vi "Tetra_RX-PROD_Close.vi"() -> (0 "error out":errorcluster={"status"=FALSE, "code"=1073676418, "source"="VISA Close in Tetra_RX-PROD_Close.vi"}, 2 "Status":string="Setting up Power Supplies...ERROR!...\rDone !!!\n...Shut Off RF\rDONE!!!")   [LabVIEW 2018]
uses:
  <vilib>/Utility/error.llb/DialogType.ctl
  Infrastructure/Test Parameter Globals_1.0.0.vi
  Initialize References/Station References Global.vi
  Tetra_Globals.vi
  Instruments/Keysight N6700/Agilent N6700 Series/Agilent N6700 Series.lvlib
  Instruments/PNA/lib functions/Agilent ENA Series.lvlib
panel:
  out "Capture RxData":bool
  out "DeleteDir(t)":bool
  out "ZipCaptures(t)":bool
  out "stripped path":path=path "C:/RageATE Results/REV-B_TETRA_RX-PROD/5_25_2022/REV-B_TETRA_RX-PROD_SN_ RGE2100033_052522-171445_RxCaptureFiles - Copy"
  in  "close serial(t)":bool=TRUE
  in  "Close Oven(t)":bool=TRUE
  out "Use PS1-2":bool=TRUE
  out "PS1-2(A)":dbl
  out "PS1-2(V)":dbl=1000000.0
  out "Use PS1-1":bool=TRUE
  out "Text":refnum<vi>
  in  "Close  PNA (T)":bool=TRUE
  in  "Close Power Supply (T)":bool=TRUE
  in  "error in (no error)":errorcluster
  out "PS1-1(A)":dbl
  out "PS1-1(V)":dbl=3.0
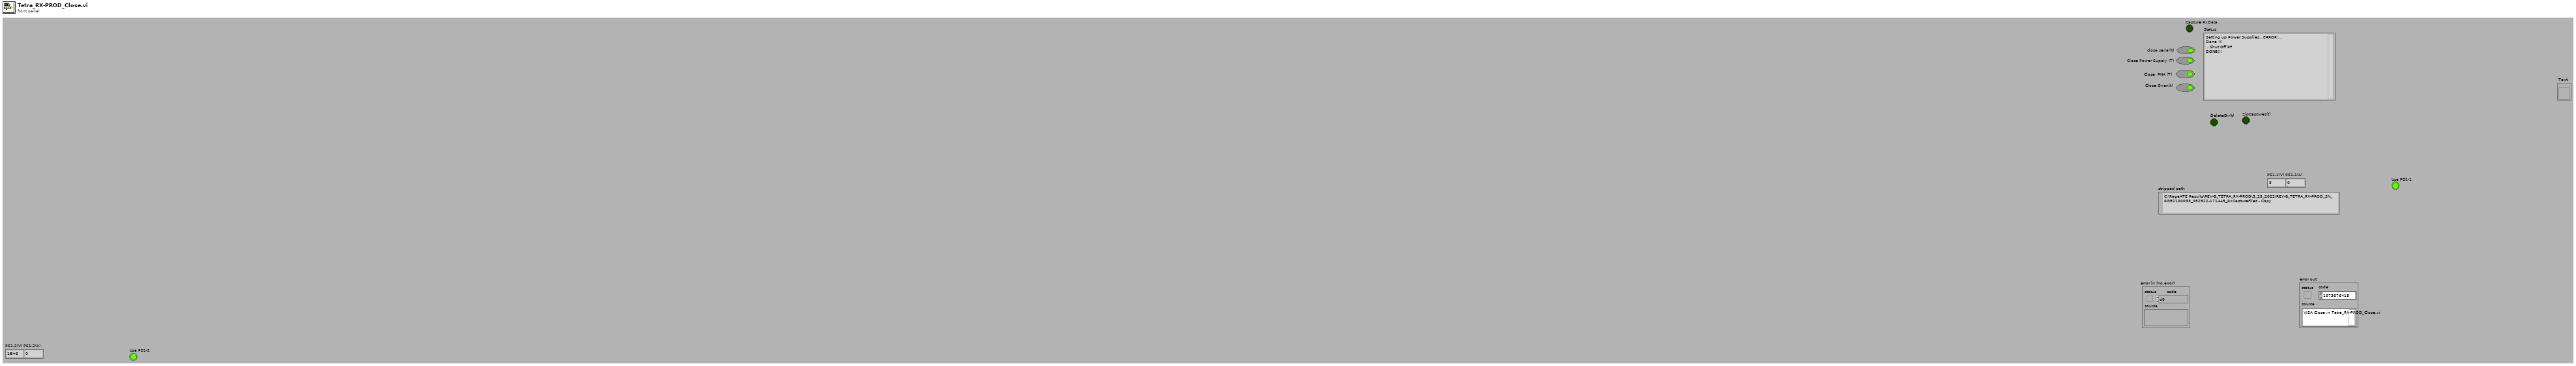
[diagram p1: front panel]
types:
  T1 = typedef "DialogType.ctl" = u16
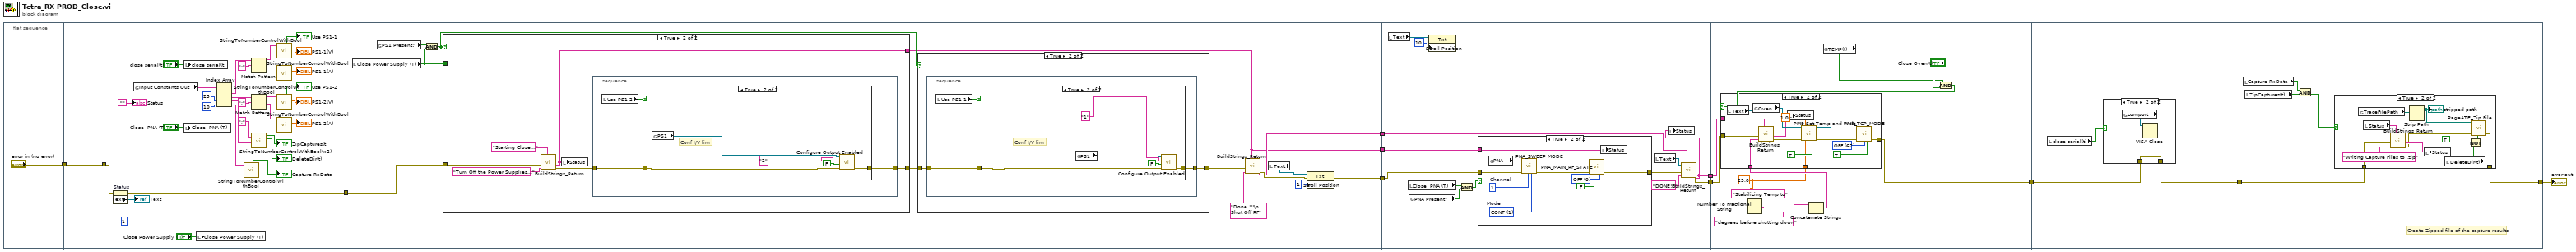
[diagram p0: block diagram]
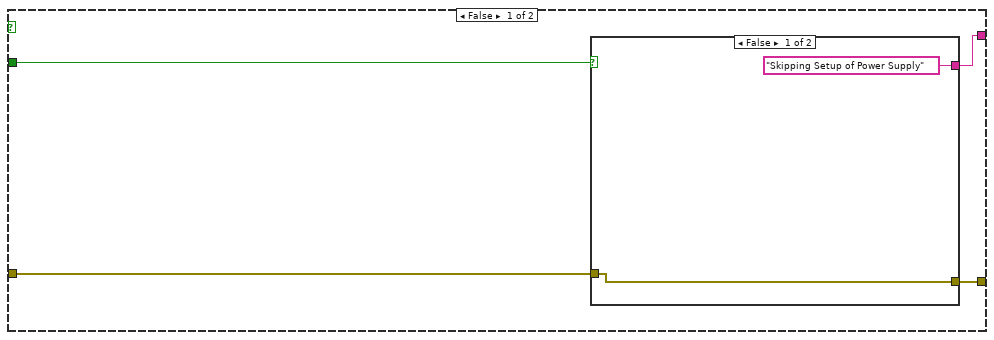
[diagram p4: hidden frame]
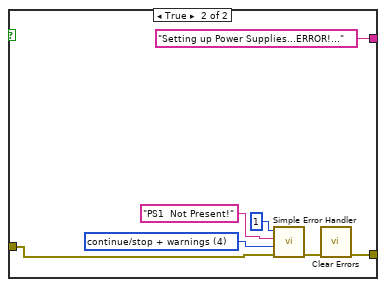
[diagram p5: hidden frame]
diagram:
  n1 = flat-sequence {
    tunnel: ["error in (no error)"] -> w5
    tunnel: w5 -> [w13]
    tunnel: [w13] -> w4
    tunnel: [w33] -> w10
    tunnel: w4 -> [w23]
    tunnel: [w56] -> w6
    tunnel: w10 -> [w52]
    tunnel: [w45] -> w3
    tunnel: [w44] -> w2
    tunnel: [w99] -> w7
    tunnel: [w108] -> w9
    tunnel: w6 -> [w102]
    tunnel: w3 -> [w100]
    tunnel: w2 -> [w98]
    tunnel: w9 -> [w128]
    tunnel: [w123] -> w8
    tunnel: w7 -> [w127]
    tunnel: w8 -> [w150]
    tunnel: [w149] -> w1
    tunnel: [w157] -> w11
    tunnel: w1 -> [w158]
    frame #0 {
    }
    frame #1 {
    }
    frame #2 {
      (unwired) u32 1 ("Text.Scroll Position")
      n2 = property on="Status" class="Str"(error in=w23) -> (error out=w33:errorcluster, "Text"=→"Text":refnum<vi>)  [unwired: 1 in, 1 out]
      n3 = global read "Test Parameter Globals_1.0.0.vi" "Input Constants Out"() -> (w24:string[])
      n4 = local write "close serial(t)"("close serial(t)") -> ()
      n5 = local write "Close  PNA (T)"("Close  PNA (T)") -> ()
      n6 = local write "Close Power Supply (T)"("Close Power Supply (T)") -> ()
      n7 = Index Array(array=w24, index #3=25 ("index"), index #4=10 ("index")) -> (element #1=w32:string, element #2=w25:string, element #3=w20:string, element #4=w15:string)  [unwired: 2 in]
      n8 = call "StringToNumberControlWithBool.vi"("String In"=w15) -> ("NOT = 0"=→"Capture RxData":bool)  [unwired: 7 in, 1 out]
      n9 = Match Pattern(string=w32, regular expression=";") -> (before substring=w38:string, after substring=w37:string)  [unwired: 1 in, 2 out]
      n10 = Match Pattern(string=w25, regular expression=";") -> (before substring=w30:string, after substring=w29:string)  [unwired: 1 in, 2 out]
      n11 = call "StringToNumberControlWithBool(x2).vi"("Seperator"=";", "string"=w20) -> ("NOT_0(2)"=→"DeleteDir(t)":bool, "NOT_0?"=→"ZipCaptures(t)":bool)  [unwired: 3 in, 5 out]
      n12 = call "StringToNumberControlWithBool.vi"("String In"=w38) -> ("Number Out"=→"PS1-1(V)":dbl, "NOT = 0"=→"Use PS1-1":bool)  [unwired: 7 in]
      n13 = call "StringToNumberControlWithBool.vi"("String In"=w37) -> ("Number Out"=→"PS1-1(A)":dbl)  [unwired: 7 in, 1 out]
      n14 = call "StringToNumberControlWithBool.vi"("String In"=w30) -> ("Number Out"=→"PS1-2(V)":dbl, "NOT = 0"=→"Use PS1-2":bool)  [unwired: 7 in]
      n15 = call "StringToNumberControlWithBool.vi"("String In"=w29) -> ("Number Out"=→"PS1-2(A)":dbl)  [unwired: 7 in, 1 out]
      "Status" <- ""
    }
    frame #3 {
      n16 = local read "Close Power Supply (T)"() -> (w46:bool)
      n17 = global read "Station References Global.vi" "PS1 Present?"() -> (w51:bool)
      n18 = And(x=w51, y=w46) -> (x .and. y?=w48:bool)
      n19 = case shown="True" w48 {
        tunnel: [w72 w83] -> w49
        tunnel: w52 -> [w71 w85]
        tunnel: [w70 w82] -> w44
        tunnel: w46 -> [w69 _]
        frame False {
          n20 = case shown="False" w69 {
            tunnel: [w74 w77] -> w72
            tunnel: w71 -> [w74 w76]
            tunnel: ["Skipping Setup of Power Supply" "Setting up Power Supplies...ERROR!..."] -> w70
            frame False {
            }
            frame True {
              w79 = T1 4 items=["no dialog", "OK message", "continue or stop message", "OK message + warnings", "continue/stop + warnings"] ("type of dialog (OK msg:1)")
              n21 = call <vilib>:"Simple Error Handler.vi"("error code (no error:0)"=1, "error source (\" \")"="PS1  Not Present!" ("error source (\" \")"), "type of dialog (OK msg:1)"=w79, "error in (no error)"=w76) -> ("error out"=w78:errorcluster)  [unwired: 1 in, 4 out]
              n22 = call <vilib>:"Clear Errors.vi"("error in (no error)"=w78) -> ("error out"=w77:errorcluster)  [unwired: 5 in, 1 out]
            }
          }
        }
        frame True {
          n23 = call "BuildStrings_Return.vi"("Input String"="Starting Close...", "New String"="Turn Off the Power Supplies...", "error in (no error)"=w85) -> ("error out"=w84:errorcluster, "concatenated string"=w82:string)  [unwired: 6 in, 1 out]
          n24 = local write "Status"(w82) -> ()
          n25 = stacked-sequence {
            tunnel: w84 -> [w90]
            tunnel: [w88] -> w83
            frame #0 {
              n26 = local read "Use PS1-2"() -> (w89:bool)
              n27 = case shown="True" w89 {
                tunnel: [w91 w94] -> w88
                tunnel: w90 -> [w91 w93]
                frame False {
                }
                frame True {
                  # "Conf I/V lim"
                  n28 = global read "Station References Global.vi" "PS1"() -> (w92:refnum<visa-resource-name>)
                  n29 = call "Configure Output Enabled.vi"("error in (no error)"=w93, "Enable Output (False)"=FALSE, "Channel Name (1)"="2", "VISA resource name"=w92) -> ("error out"=w94:errorcluster)  [unwired: 6 in, 1 out]
                }
              }
            }
          }
        }
      }
      n30 = case shown="True" w48 {
        tunnel: [w57 w59] -> w47
        tunnel: w49 -> [w57 w58]
        frame False {
        }
        frame True {
          n31 = stacked-sequence {
            tunnel: w58 -> [w62]
            tunnel: [w60] -> w59
            frame #0 {
              n32 = local read "Use PS1-1"() -> (w61:bool)
              n33 = case shown="True" w61 {
                tunnel: [w63 w66] -> w60
                tunnel: w62 -> [w63 w65]
                frame False {
                }
                frame True {
                  # "Conf I/V lim"
                  n34 = global read "Station References Global.vi" "PS1"() -> (w64:refnum<visa-resource-name>)
                  n35 = call "Configure Output Enabled.vi"("error in (no error)"=w65, "Enable Output (False)"=FALSE, "Channel Name (1)"="1", "VISA resource name"=w64) -> ("error out"=w66:errorcluster)  [unwired: 6 in, 1 out]
                }
              }
            }
          }
        }
      }
      n36 = call "BuildStrings_Return.vi"("Input String"=w44, "New String"="Done !!!\n...Shut Off RF", "error in (no error)"=w47) -> ("error out"=w53:errorcluster, "concatenated string"=w45:string)  [unwired: 6 in, 1 out]
      n37 = local read "Text"() -> (w55:refnum<vi>)
      n38 = property class="Txt"(reference=w55, error in=w53, "Scroll Position"=u32 1) -> (error out=w56:errorcluster)  [unwired: 1 out]
    }
    frame #4 {
      n39 = local read "Text"() -> (w106:refnum<vi>)
      n40 = local read "Close  PNA (T)"() -> (w105:bool)
      n41 = global read "Station References Global.vi" "PNA Present?"() -> (w104:bool)
      n42 = property class="Txt"(reference=w106, "Scroll Position"=u32 10) -> ()  [unwired: 1 in, 2 out]
      n43 = And(x=w105, y=w104) -> (x .and. y?=w103:bool)
      n44 = case shown="True" w103 {
        tunnel: w102 -> [w110 w118]
        tunnel: [w110 w116] -> w101
        tunnel: w98 -> [_ w111]
        frame False {
        }
        frame True {
          w113 = 0 items=["OFF", "ON"] ("STATE(0=OFF)")
          w119 = 1 items=["HOLD", "CONT", "GROUP", "SINGLE"]  # Mode
          w120 = 1  # Channel
          n45 = global read "Station References Global.vi" "PNA"() -> (w117:refnum<visa-resource-name>)
          n46 = call "PNA_SWEEP MODE.vi"("Mode"=w119, "Channel"=w120, "error in (no error)"=w118, "VISA resource name"=w117) -> ("error out"=w115:errorcluster, "VISA resource name out"=w114:refnum<visa-resource-name>)  [unwired: 6 in]
          n47 = call "PNA_MAIN_RF_STATE.vi"("Session In"=w114, "error in"=w115, "RO(T)"=FALSE, "STATE(0=OFF)"=w113) -> ("error out"=w116:errorcluster)  [unwired: 9 in, 2 out]
          n48 = local write "Status"(w111) -> ()
        }
      }
      n49 = local read "Text"() -> (w97:refnum<vi>)
      n50 = call "BuildStrings_Return.vi"("Input String"=w100, "New String"="DONE!!!", "error in (no error)"=w101, "reference"=w97) -> ("error out"=w108:errorcluster, "concatenated string"=w99:string)  [unwired: 5 in, 1 out]
      n51 = local write "Status"(w99) -> ()
    }
    frame #5 {
      w121 = 25.0 ("Set Point")
      n52 = Number To Fractional String(number=w121) -> (F-format string=w122:string)  [unwired: 3 in]
      n53 = Concatenate Strings("Stabilizing Temp to" ("New String"), w122, "degrees before shutting down" ("string")) -> (w126:string)
      n54 = global read "Tetra_Globals.vi" "TEMP(t)"() -> (w125:bool)
      n55 = And(x=w125, y="Close Oven(t)") -> (x .and. y?=w124:bool)
      n56 = case shown="True" w124 {
        tunnel: w128 -> [w132 w144]
        tunnel: w127 -> [_ w146]
        tunnel: w126 -> [_ w145]
        tunnel: [w132 w137] -> w123
        tunnel: w121 -> [_ w134]
        frame False {
        }
        frame True {
          w139 = u16 62 items=["READ ONLY"=0, "AUTO"=10, "OFF"=62, "MAN"=54] ("MODE")
          n57 = local read "Text"() -> (w135:refnum<vi>)
          n58 = global read "Station References Global.vi" "Oven"() -> (w147:refnum<visa-resource-name>)
          n59 = call "BuildStrings_Return.vi"("Input String"=w146, "New String"=w145, "error in (no error)"=w144, "reference"=w135) -> ("error out"=w143:errorcluster, "concatenated string"=w141:string)  [unwired: 5 in, 1 out]
          n60 = local write "Status"(w141) -> ()
          n61 = call "PM9 Set Temp and Wait.vi"("VISA"=w147, "Error In"=w143, "Accuracy +/-"=1.0, "Set Point"=w134, "close session(t)"=TRUE) -> ("visa"=w136:refnum<visa-resource-name>, "error out"=w140:errorcluster)  [unwired: 11 in, 2 out]
          n62 = call "PM9_TCP_MODE.vi"("VISA"=w136, "error in (no error)"=w140, "MODE"=w139, "Close tcp(t)"=TRUE) -> ("error out"=w137:errorcluster)  [unwired: 8 in, 3 out]
        }
      }
    }
    frame #6 {
      n63 = local read "close serial(t)"() -> (w148:bool)
      n64 = case shown="True" w148 {
        tunnel: w150 -> [w151 w152]
        tunnel: [w151 w152] -> w149
        frame False {
        }
        frame True {
          n65 = global read "Tetra_Globals.vi" "comport"() -> (w153:refnum<visa-resource-name>)
          n66 = VISA Close(VISA resource name=w153) -> ()  [unwired: 1 in, 1 out]
        }
      }
    }
    frame #7 {
      # "Create Zipped file of the capture results"
      n67 = local read "Capture RxData"() -> (w154:bool)
      n68 = local read "ZipCaptures(t)"() -> (w156:bool)
      n69 = And(x=w154, y=w156) -> (x .and. y?=w155:bool)
      n70 = case shown="True" w155 {
        tunnel: w158 -> [w159 w166]
        tunnel: [w159 w162] -> w157
        frame False {
        }
        frame True {
          (unwired) TRUE ("PreserveOrigFolder(t)")
          n71 = global read "Tetra_Globals.vi" "TraceFilePath"() -> (w169:path)
          n72 = local read "Status"() -> (w167:string)
          n73 = call "BuildStrings_Return.vi"("Input String"=w167, "New String"="Writing Capture Files to .zip", "error in (no error)"=w166) -> ("error out"=w163:errorcluster, "concatenated string"=w164:string)  [unwired: 6 in, 1 out]
          n74 = Strip Path(path=w169) -> (stripped path=w168:path)  [unwired: 1 out]
          "stripped path" <- w168
          n75 = local write "Status"(w164) -> ()
          n76 = local read "DeleteDir(t)"() -> (w161:bool)
          n77 = Not(x=w161) -> (.not. x?=w160:bool)
          n78 = call "RageATE_Zip File.vi"("input path"=w168, "error in"=w163, "PreserveOrigFolder(t)"=w160) -> ("error out"=w162:errorcluster)  [unwired: 10 in, 2 out]
        }
      }
    }
  }
  "error out" <- w11
